vi "Prepare Control.vi"(7 "VolatusAPI":refnum<class "VolatusAPI.lvclass">, 8 "error in (no error)":errorcluster, 11 "PulsedValve in":refnum<class "PulsedControl.lvclass">) -> (0 "error out":errorcluster, 3 "PulsedValve out":refnum<class "PulsedControl.lvclass">)   [LabVIEW 2020, in "VolatusControl.lvlib" / "PulsedControl.lvclass"]
uses:
  PulsedControl.lvclass
  PulsedControl.lvclass/PulsedControl.ctl
  Volatus/VolatusAPI/VolatusAPI.lvclass
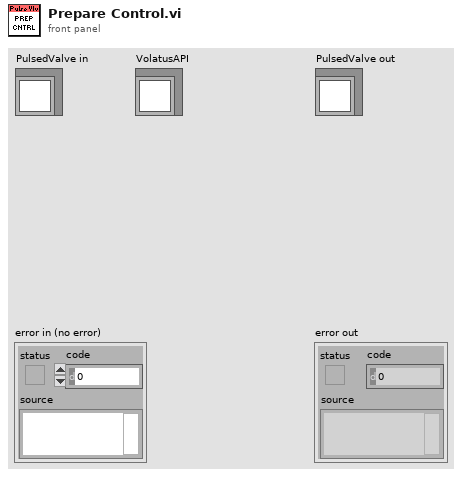
[diagram p1: front panel]
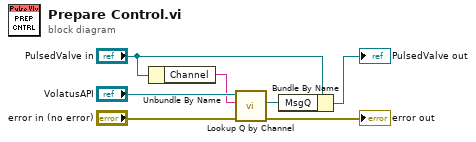
[diagram p0: block diagram]
diagram:
  n1 = Unbundle By Name("PulsedValve in") -> ("Channel"=w5:string)
  n2 = call "Lookup Q by Channel.vi"("error in (no error)"="error in (no error)", "Channel Name"=w5, "VolatusAPI in"="VolatusAPI") -> ("error out"=→"error out":errorcluster, "MessageQ"=w3:refnum<class "MessageQ.lvclass">)  [unwired: 6 in, 1 out]
  n3 = Bundle By Name(cluster="PulsedValve in", "MsgQ"=w3) -> (→"PulsedValve out":refnum<class "PulsedControl.lvclass">)
